vi "Data_Path_Of_Day.vi"(8 "error in (no error)":errorcluster, 11 "SOFTWARE Inputs":T1={"Application Directory"=path "D:/S.O.F.T.S/LABVIEW/PIL", "Software Version"="1.0.0", "Data Path"=path "D:/PIRENEA/DATA", "XML Path"=path "D:/PIRENEA/DATA", "XML File Filter"="*.xml", "XML Saved Path"=path "D:/S.O.F.T.S/LABVIEW/PIL/resources", "Excit Scripts Path"=path "D:/PIRENEA/EXCIT_SCRIPTS", "Excit Scripts File Filter"="*.txt", "Excit Waveforms Path"=path "D:/PIRENEA/EXCIT_WFMS", "Excit Waveforms File Filter"="*.bin", "Timing Scripts Path"=path "D:/PIRENEA/TIMING_SCRIPTS", "Timing Scripts File Filter"="*.txt", "Timing Waveforms Path"=path "D:/PIRENEA/TIMING_WFMS", "Timing Waveforms File Filter"="*.bin", "Trapping Waveforms Path"=path "D:/PIRENEA/TRAPPING_WFMS", "Trapping Waveforms File Filter"="*.bin"}) -> (0 "error out":errorcluster caption="sortie d'erreur", 3 "Path of the Day":path)   [LabVIEW 2018]
doc: "This VI returns the PATH of the day for the data, with the naming convention :\nDATA_PATH\\yyyy\\data_yyyy_mm_dd\\yyyy_mm_dd"
uses:
  controls/SOFTWARE_Inputs.ctl
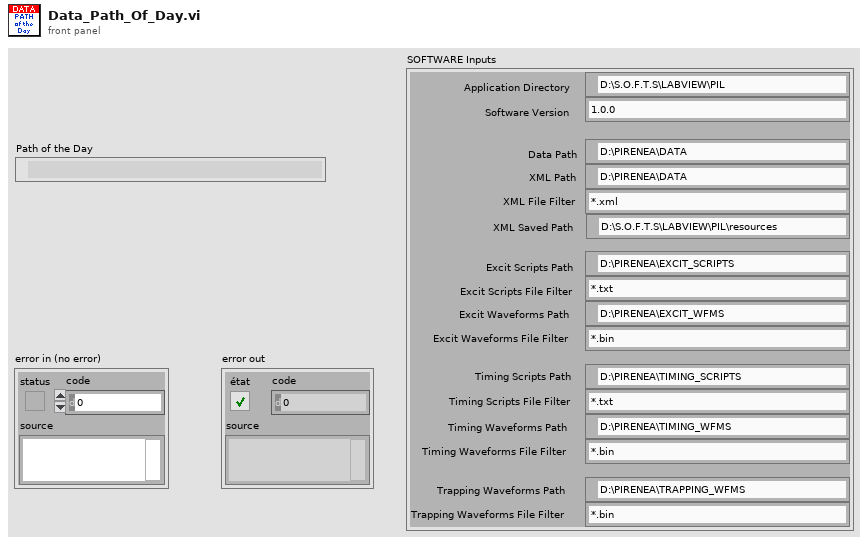
[diagram p1: front panel]
types:
  T1 = typedef "SOFTWARE_Inputs.ctl" = cluster{"Application Directory":path, "Software Version":string, "Data Path":path, "XML Path":path, "XML File Filter":string, "XML Saved Path":path, "Excit Scripts Path":path, "Excit Scripts File Filter":string, "Excit Waveforms Path":path, "Excit Waveforms File Filter":string, "Timing Scripts Path":path, "Timing Scripts File Filter":string, "Timing Waveforms Path":path, "Timing Waveforms File Filter":string, "Trapping Waveforms Path":path, "Trapping Waveforms File Filter":string}
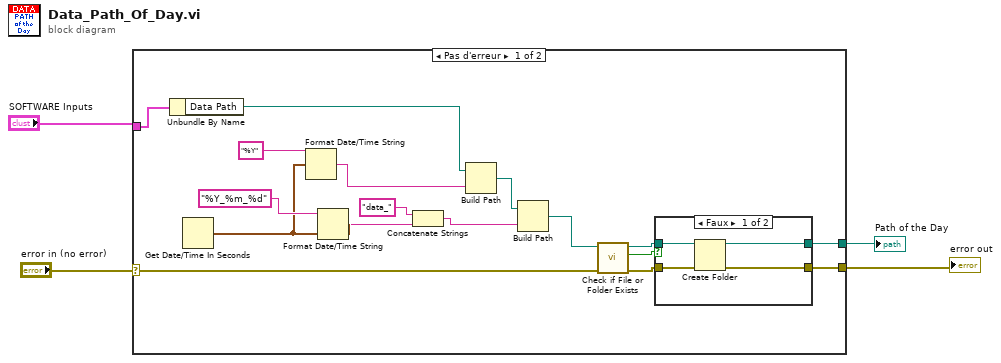
[diagram p0: block diagram]
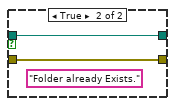
[diagram p2: hidden frame]
diagram:
  n1 = case shown="Pas d'erreur" "error in (no error)" {
    selector: "error in (no error)" -> [w5 w28]
    tunnel: "SOFTWARE Inputs" -> [w13 _]
    tunnel: [w11 w28] -> w3
    tunnel: [w6 _] -> w2
    frame No Error {
      n2 = Unbundle By Name(w13) -> ("Data Path"=w12:path)
      n3 = Get Date/Time In Seconds() -> (seconds since 1Jan1904=w20:timestamp)
      n4 = Format Date/Time String(time format string (%c)="%Y" ("chaîne de format de l'heure (%c)"), seconds (now)=w20) -> (date/time string=w18:string)  [unwired: 1 in]
      n5 = Format Date/Time String(time format string (%c)="%Y_%m_%d" ("chaîne de format de l'heure (%c)"), seconds (now)=w20) -> (date/time string=w7:string)  [unwired: 1 in]
      n6 = Concatenate Strings("data_" ("chaîne"), w7) -> (w8:string)
      n7 = Build Path(base path=w12, name or relative path=w18) -> (appended path=w17:path)
      n8 = Build Path(base path=w17, name or relative path=w8) -> (appended path=w10:path)
      n9 = call <vilib>:"Check if File or Folder Exists.vi"("error in (no error)"=w5, "path"=w10) -> ("error out"=w14:errorcluster, "file or folder exists?"=w16:bool, "dup path"=w15:path)  [unwired: 7 in]
      n10 = case shown="Faux" w16 {
        tunnel: w15 -> [w25 w27]
        tunnel: w14 -> [w24 w26]
        tunnel: [w23 w27] -> w6
        tunnel: [w22 w26] -> w11
        frame False {
          n11 = Create Folder(path (use dialog)=w25, error in=w24) -> (created path=w23:path, error out=w22:errorcluster)  [unwired: 1 in, 1 out]
        }
        frame True {
          (unwired) "Folder already Exists." ("Created Path")
        }
      }
    }
    frame Error {
    }
  }
  "error out" <- w3
  "Path of the Day" <- w2
